vi "gxml_UnescapeChar.vi"(10 "XML In":string) -> (2 "XML Out":string)   [LabVIEW 2011, in "Third Party VIs.lvlib" / "GXML.lvlib"]
doc: "This VI unescapes all characters with decimal codes between 128 and 255 that have been escaped to &#nnn; (nnn is the character decimal code)"
uses:
  GXML.lvlib
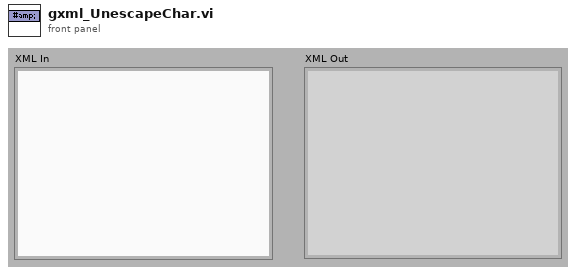
[diagram p1: front panel]
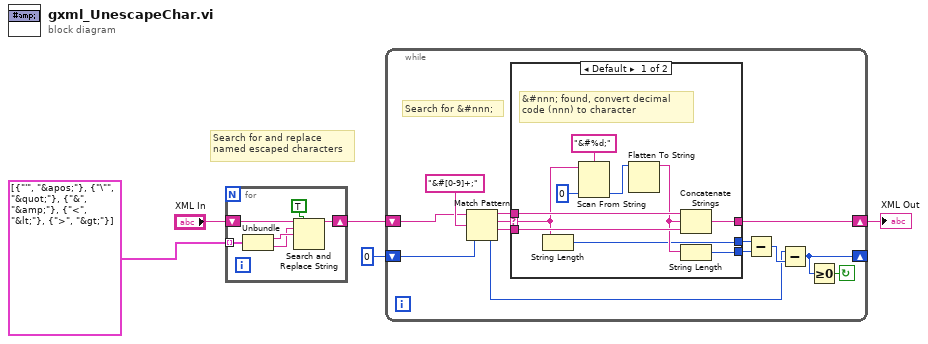
[diagram p0: block diagram]
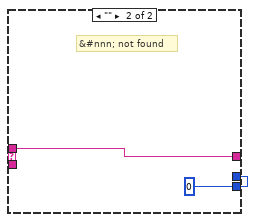
[diagram p2: hidden frame]
diagram:
  # "Search for and replace\nnamed escaped characters"
  n1 = for {
    shift-right: [w9] -> w2
    shift-left: "XML In" -> [w10]
    tunnel: cluster{string, string}[] [{"'", "&apos;"}, {"\"", "&quot;"}, {"&", "&amp;"}, {"<", "&lt;"}, {">", "&gt;"}] -> [w8] mode=indexing
    n2 = Unbundle(w8) -> (w7:string, w6:string)
    n3 = Search and Replace String(replace all?=TRUE ("replace all? (F)"), input string=w10, search string=w6, replace string=w7) -> (result string=w9:string)  [unwired: 4 in, 3 out]
  }
  n4 = while {
    shift-left: 0 -> [w23]
    shift-right: [w13] -> _
    shift-left: w2 -> [w12]
    shift-right: [w19] -> w4
    stop <- w18 continue-if-true
    # "Search for &#nnn;"
    n5 = Match Pattern(string=w12, regular expression="&#[0-9]+;", offset (0)=w23) -> (before substring=w21:string, match substring=w22:string, after substring=w20:string, offset past match=w14:i32)
    n6 = case shown="Default" w22 {
      selector: w22 -> [w27 _]
      tunnel: w21 -> [w33 w36]
      tunnel: w20 -> [w31 _]
      tunnel: [w32 w36] -> w19
      tunnel: [w29 w35] -> w16
      tunnel: [w34 w35] -> w15
      frame Default {
        # "&#nnn; found, convert decimal \ncode (nnn) to character"
        n7 = String Length(string=w27) -> (length=w29:i32)
        n8 = Scan From String(format string="&#%d;" ("Input String"), input string=w27, default 1=u8 0) -> (output 1=w26:u8)  [unwired: 2 in, 3 out]
        n9 = Flatten To String(anything=w26) -> (data string=w30:string)  [unwired: 3 in, 2 out]
        n10 = Concatenate Strings(w33, w30, w31) -> (w32:string)
        n11 = String Length(string=w30) -> (length=w34:i32)
      }
      frame "" {
        w35 = 0
        # "&#nnn; not found"
      }
    }
    n12 = Subtract(x=w16, y=w15) -> (x-y=w17:i32)
    n13 = Subtract(x=w14, y=w17) -> (x-y=w13:i32)
    n14 = Greater Or Equal To 0?(x=w13) -> (x >= 0?=w18:bool)
  }
  "XML Out" <- w4
